vi "Open and Stop MV.vi"(7 "init":bool, 8 "error in (no error)":errorcluster, 11 "Stand in":refnum<class "Stand.lvclass">) -> (0 "error out":errorcluster)   [LabVIEW 2019, in "Stand.lvclass"]
uses:
  Stand.lvclass
  Stand.lvclass/Stand.ctl
  dY_dX_Calculator/delayValue.lvclass/delayValue.ctl
  NeedleValve_class/Cmd.ctl
  dY_dX_Calculator/delayValue.lvclass
  NeedleValve_class/NeedleValve.lvclass
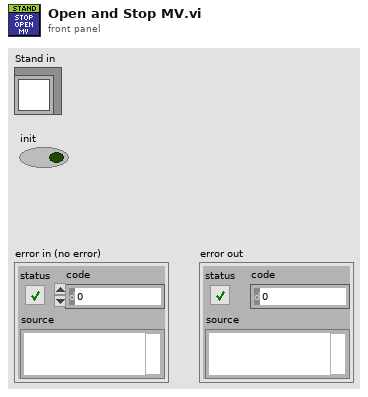
[diagram p1: front panel]
types:
  T1 = typedef "Direction.ctl" = enum8{"DUT", "Chamber"}
  T2 = typedef "NeedleValve.lvclass/Cmd.ctl" = enum16{"Open", "Close", "Stop", "Prep open"}
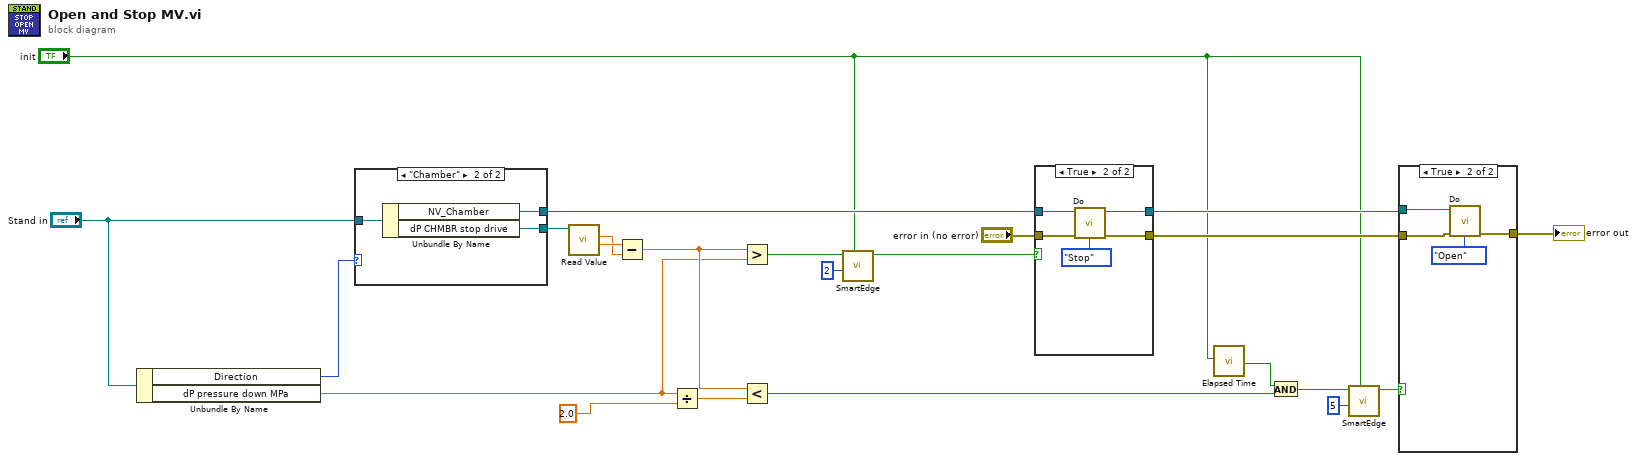
[diagram p0: block diagram]
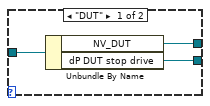
[diagram p4: hidden frame]
diagram:
  n1 = Unbundle By Name("Stand in") -> ("Direction"=w4:T1, "dP pressure down MPa"=w9:dbl)
  n2 = case shown="\"Chamber\"" w4 {
    tunnel: [w26 w29] -> w7
    tunnel: [w25 w28] -> w12
    tunnel: "Stand in" -> [w24 w27]
    frame "DUT" {
      n3 = Unbundle By Name(w24) -> ("NV_DUT"=w25:refnum<class "NeedleValve.lvclass">, "dP DUT stop drive"=w26:refnum<class "delayValue.lvclass">)
    }
    frame "Chamber" {
      n4 = Unbundle By Name(w27) -> ("NV_Chamber"=w28:refnum<class "NeedleValve.lvclass">, "dP CHMBR stop drive"=w29:refnum<class "delayValue.lvclass">)
    }
  }
  n5 = call "Read Value.vi"("dY_dX_Calculator in"=w7) -> ("oldValue"=w6:dbl, "currValue"=w5:dbl)  [unwired: 9 in]
  n6 = Subtract(x=w6, y=w5) -> (x-y=w15:dbl)
  n7 = Divide(x=w9, y=2.0) -> (x/y=w14:dbl)
  n8 = Greater?(x=w15, y=w9) -> (0:w10:bool)
  n9 = Less?(x=w15, y=w14) -> (x < y?=w17:bool)
  n10 = call "SmartEdge.vi"("init"="init", "Filter Length"=2, "in"=w10) -> ("edge"=w11:bool)  [unwired: 8 in]
  n11 = case shown="True" w11 {
    tunnel: [w30 w36] -> w16
    tunnel: [w31 w34] -> w13
    tunnel: w12 -> [w31 w33]
    tunnel: "error in (no error)" -> [w30 w32]
    frame False {
    }
    frame True {
      n12 = call "Do.vi"("Cmd"=Cmd."Stop", "error in (no error)"=w32, "NeedleValve in"=w33) -> ("error out"=w36:errorcluster, "NeedleValve out"=w34:refnum<class "NeedleValve.lvclass">)  [unwired: 7 in]
    }
  }
  n13 = call "Elapsed Time"("Reset"="init") -> ("Time has Elapsed"=w2:bool)  [unwired: 11 in, 7 out]
  n14 = And(x=w2, y=w17) -> (x .and. y?=w3:bool)
  n15 = call "SmartEdge.vi"("init"="init", "Filter Length"=5, "in"=w3) -> ("edge"=w18:bool)  [unwired: 8 in]
  n16 = case shown="True" w18 {
    tunnel: [w37 w41] -> w19
    tunnel: w13 -> [_ w39]
    tunnel: w16 -> [w37 w38]
    frame False {
    }
    frame True {
      n17 = call "Do.vi"("Cmd"=Cmd."Open", "error in (no error)"=w38, "NeedleValve in"=w39) -> ("error out"=w41:errorcluster)  [unwired: 7 in, 1 out]
    }
  }
  "error out" <- w19
